vi "Stream Begin All Sensors.vi"(8 "error in":errorcluster, 11 "UART port in":T1) -> (0 "error out":errorcluster, 3 "UART port out":T1)   [LabVIEW 2014]
doc: "Begin a sensor stream containing all iRobot Create sensor data. After this command is issued, the iRobot Create should begin sending packets containing all sensor data.\n\nThis VI both writes to AND reads from the serial port."
uses:
  Advanced/UART/iRobot UART Port Type.ctl
  Sensor ID.ctl
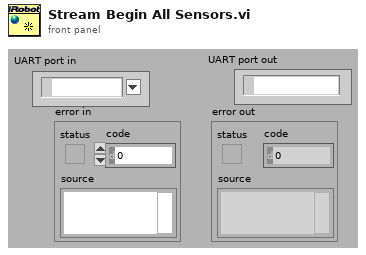
[diagram p1: front panel]
types:
  T1 = typedef "iRobot UART Port Type.ctl" = refnum<visa-resource-name>
  T2 = typedef "Sensor ID.ctl" = enum8{"Sensor Group 0", "Sensor Group 1", "Sensor Group 2", "Sensor Group 3", "Sensor Group 4", "Sensor Group 5", "Sensor Group 6", "Bump + Wheel Drop", "Wall", "Cliff Left", "Cliff Front Left", "Cliff Front Right", "Cliff Right", "Virtual Wall", "Low Side Driver + Wheel Overcurrent", "Unused 0", "Unused 1", "Infrared", "Buttons", "Distance", "Angle", "Charging State", "Voltage", "Current", "Battery Temperature", "Battery Charge", "Battery Capacity", "Wall Signal", "Cliff Left Signal", "Cliff Front Left Signal", "Cliff Front Right Signal", "Cliff Right Signal", "Cargo Bay Digital Inputs", "Cargo Bay Analog Signal", "Charging Sources Available", "OI Mode", "Song Number", "Song Playing", "Number of Stream Packets", "Requested Velocity", "Requested Radius", "Requested Right Velocity", "Requested Left Velocity"}
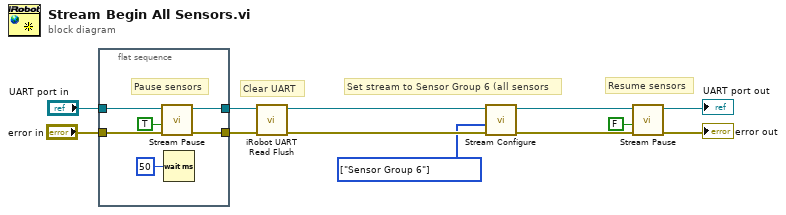
[diagram p0: block diagram]
diagram:
  w4 = T2[] [enum."Sensor Group 6"] items=["Sensor Group 0", "Sensor Group 1", "Sensor Group 2", "Sensor Group 3", "Sensor Group 4", "Sensor Group 5", "Sensor Group 6", "Bump + Wheel Drop", "Wall", "Cliff Left", "Cliff Front Left", "Cliff Front Right", "Cliff Right", "Virtual Wall", "Low Side Driver + Wheel Overcurrent", "Unused 0", "Unused 1", "Infrared", "Buttons", "Distance", "Angle", "Charging State", "Voltage", "Current", "Battery Temperature", "Battery Charge", "Battery Capacity", "Wall Signal", "Cliff Left Signal", "Cliff Front Left Signal", "Cliff Front Right Signal", "Cliff Right Signal", "Cargo Bay Digital Inputs", "Cargo Bay Analog Signal", "Charging Sources Available", "OI Mode", "Song Number", "Song Playing", "Number of Stream Packets", "Requested Velocity", "Requested Radius", "Requested Right Velocity", "Requested Left Velocity"] ("Sensors")
  # "Resume sensors"
  # "Set stream to Sensor Group 6 (all sensors"
  # "Clear UART"
  n1 = flat-sequence {
    tunnel: "UART port in" -> [w18]
    tunnel: "error in" -> [w17]
    tunnel: [w16] -> w10
    tunnel: [w15] -> w9
    frame #0 {
      # "Pause sensors"
      n2 = call "Stream Pause.vi"("error in"=w17, "Pause?"=TRUE ("Resume?"), "UART port in"=w18) -> ("error out"=w15:errorcluster, "UART port out"=w16:T1)  [unwired: 7 in]
      n3 = Wait (ms)(milliseconds to wait=u32 50) -> ()  [unwired: 1 out]
    }
  }
  n4 = call "iRobot UART Read Flush.vi"("error in"=w9, "UART port in"=w10) -> ("error out"=w7:errorcluster, "UART port out"=w8:T1)  [unwired: 7 in, 1 out]
  n5 = call "Stream Configure.vi"("error in"=w7, "Sensors"=w4, "UART port in"=w8) -> ("error out"=w5:errorcluster, "UART port out"=w6:T1)  [unwired: 7 in]
  n6 = call "Stream Pause.vi"("error in"=w5, "Pause?"=FALSE ("Resume?"), "UART port in"=w6) -> ("error out"=→"error out":errorcluster, "UART port out"=→"UART port out":T1)  [unwired: 7 in]
